vi "sub_SDR_FreqMeas.vi"(7 "Sampling Freq.":dbl, 10 "Received data in":cdb[](array[numeric])) -> (2 "Frequency Estimation":dbl)   [LabVIEW 2012]
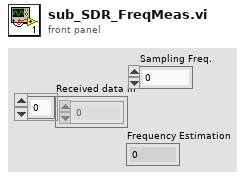
[diagram p1: front panel]
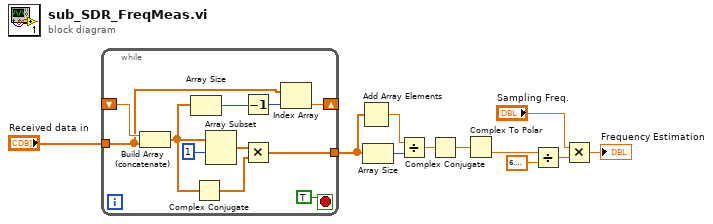
[diagram p0: block diagram]
diagram:
  n1 = while {
    tunnel: "Received data in" -> [w19]
    shift-right: [w17] -> _
    shift-left: _ -> [w21]
    tunnel: [w12] -> w8
    stop <- TRUE stop-if-true
    n2 = Build Array (concatenate)(w21, w19) -> (w15:cdb[])
    n3 = Array Size(array=w15) -> (size(s)=w20:i32)
    n4 = Complex Conjugate(1:w15) -> (0:w14:cdb[])
    n5 = Array Subset(array=w15, index=1) -> (w13:cdb[])  [unwired: 1 in]
    n6 = Decrement(x=w20) -> (x-1=w18:i32)
    n7 = Multiply(x=w13, y=w14) -> (x*y=w12:cdb[])
    n8 = Index Array(array=w19, index=w18) -> (element=w17:cdb)
  }
  n9 = Add Array Elements(numeric array=w8) -> (sum=w7:cdb)
  n10 = Array Size(array=w8) -> (size(s)=w9:i32)
  n11 = Divide(x=w7, y=w9) -> (x/y=w10:cdb)
  n12 = Complex Conjugate(1:w10) -> (0:w11:cdb)
  n13 = Complex To Polar(r * e^(i*theta)=w11) -> (theta=w5:dbl)  [unwired: 1 out]
  n14 = Divide(x=w5, y=6.283185307179586) -> (x/y=w3:dbl)
  n15 = Multiply(x="Sampling Freq.", y=w3) -> (x*y=→"Frequency Estimation":dbl)
